vi "Tree Set Default.vi"(8 "error in (no error)":errorcluster, 10 "Node":refnum<data-value>, 11 "Tree DVR in":refnum<data-value>) -> (0 "error out":errorcluster, 3 "Tree DVR out":refnum<data-value>)   [LabVIEW 2012, in "MDSplus.lvlib"]
doc: "Set the default position in the tree."
uses:
  <vilib>/MDSplus/Library/MDSplus.lvlib
  <vilib>/MDSplus/Classes/Tree_Class/Tree.lvclass
  <vilib>/MDSplus/Classes/Data_Class/TreeNode_Class/TreeNode.lvclass
panel:
  out "Node Out":refnum<data-value>
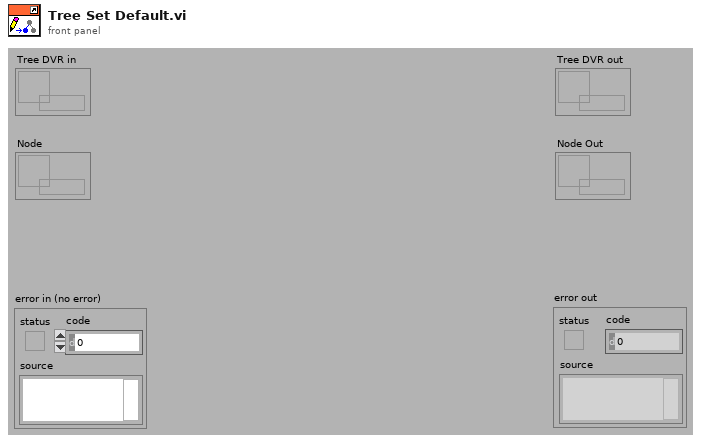
[diagram p1: front panel]
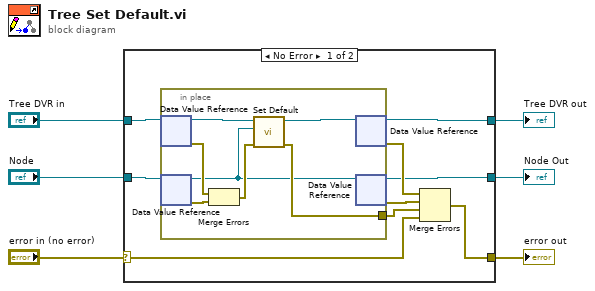
[diagram p0: block diagram]
diagram:
  n1 = case shown="No Error" "error in (no error)" {
    selector: "error in (no error)" -> [w10 w23]
    tunnel: "Tree DVR in" -> [w15 w25]
    tunnel: [w12 w23] -> w6
    tunnel: [w13 w25] -> w3
    tunnel: "Node" -> [w11 w24]
    tunnel: [w7 w24] -> w1
    frame No Error {
      n2 = in-place {
        in-place-border: [w17] -> w8
        n3 = in-place-dvr #1(w15) -> (w22:refnum<class "Tree.lvclass">, w19:errorcluster)
        n4 = in-place-dvr #2(w11) -> (w16:refnum<class "TreeNode.lvclass">, w18:errorcluster)
        n5 = Merge Errors(w19, w18) -> (w20:errorcluster)
        n6 = call-dynamic "Set Default.vi"("error in (no error)"=w20, "Node"=w16, "Tree in"=w22) -> ("error out"=w17:errorcluster, "Tree out"=w21:refnum<class "Tree.lvclass">)  [unwired: 6 in, 1 out]
        n7 = in-place-dvr #1(w21) -> (w13:refnum<data-value>, w14:errorcluster)
        n8 = in-place-dvr #2(w16) -> (w7:refnum<data-value>, w9:errorcluster)
      }
      n9 = Merge Errors(w14, w9, w8, w10) -> (w12:errorcluster)
    }
    frame Error {
    }
  }
  "error out" <- w6
  "Tree DVR out" <- w3
  "Node Out" <- w1
